vi "Send command.vi"(7 "Action":T2, 8 "error in (no error)":errorcluster, 9 "Set Values in":T1, 10 "d(0.0)":dbl, 11 "VISA resource":refnum<visa-resource-name>) -> (0 "error out":errorcluster, 1 "Set Values":T1, 3 "VISA resource out":refnum<visa-resource-name>)   [LabVIEW 2011]
doc: "Sends the actual command values, waits for the return strnig, but does not interprate it."
uses:
  Magna Commands.ctl
  Magna Configuration Values Set.ctl
  Magna PSU.lvlib
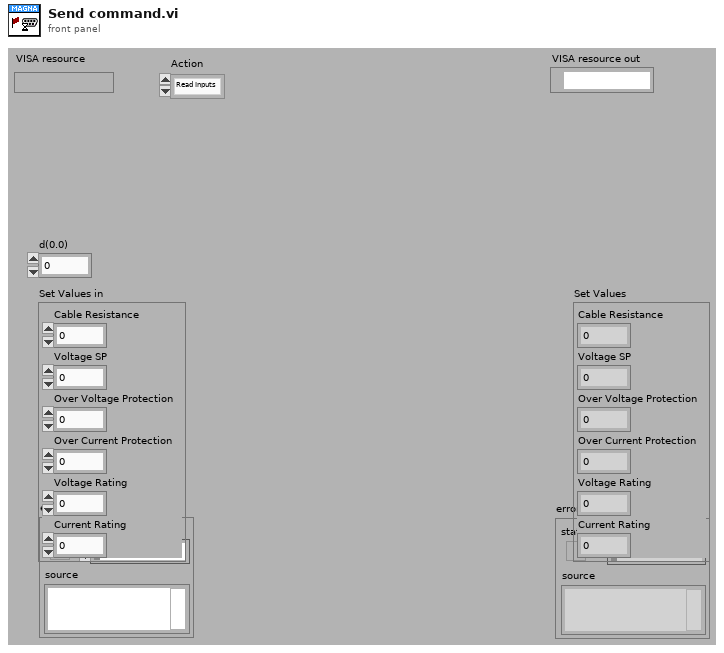
[diagram p1: front panel]
types:
  T1 = typedef "Magna Configuration Values Set.ctl" = cluster{"Cable Resistance":dbl, "Voltage SP":dbl, "Over Voltage Protection":dbl, "Over Current Protection":dbl, "Voltage Rating":dbl, "Current Rating":dbl}
  T2 = typedef "Magna Commands.ctl" = enum16{"Read Inputs", "HV ON", "HV OFF", "Set Resistance", "Set Head Voltage SP"}
  T3 = typedef "Options  All pages and custom.ctl" = cluster{"P 1 (App)":T4, "P 2":T5, "P 3":T6, "P 4":T9, "P 5":T14, "P 6 (Err)":T15, "P 7 (Expert)":T16, "P 8 (Depth)":T18, "C 1":T19, "C 2":T20}
  T4 = typedef "Options Page 1 (App).ctl" = cluster{"Result files":path, "PCP Interface":string, "Tractor/Stroker Interface":string, "Tractor Interface":string, "Modem Status Interface":string, "Audible Alarm":bool, "Force alarm on Technical":bool, "Force alarm on HH":bool, "Force alarm on LL":bool, "Force alarm on H":bool, "Force alarm on L":bool}
  T5 = typedef "Options Page 2.ctl" = cluster{"Solenoid & Relay latching time":u16, "Tractor relay 1":dbl, "Tractor relay 2":dbl, "Tractor Solenoid limit":dbl}
  T6 = typedef "Options Page 3.ctl" = cluster{"Min resistance":dbl, "Max resistance":dbl, "Head voltage range":T7, "Max voltage jump":dbl, "Maximum resistance change":dbl, "Start Telemetry Voltage":dbl, "Start Telemetry Timeout":dbl, "Start Motor Voltage":dbl, "Stop Motor Voltage":dbl, "Pass Mode Warning Voltage":dbl, "Relay Switch Voltage":dbl, "Relay Status Loss Voltage":dbl, "Samples to average":i32, "PSU type DO NOT USE":T8, "Magna OVP":dbl, "Magna Current Limit":dbl}
  T7 = typedef "PCP type List.ctl" = enum16{"0 - 350V", "0 - 450V", "0 - 600V"}
  T8 = typedef "PSU Type.ctl" = enum16{"Unipower", "Magna 8.3A", "Magna 12A", "None"}
  T9 = typedef "Options Page 4.ctl" = cluster{"Solenoid & Relay latching time":u16, "Stroker relay 1":dbl, "Stroker Relay 2":dbl, "Stroker Solenoid limit":dbl, "Force det.":T10, "Stroke force lim.":dbl, "Anchor Enabled Pressure":dbl, "Tacometer puls":dbl, "Default anchor behavior":T11, "Default stroker behavior":T12, "Default stroker force limit (tonne)":dbl, "Slips Size":T13}
  T10 = typedef "Stroke force selector.ctl" = enum16{"Stroke in = node 1", "Strok out = node 1"}
  T11 = typedef "Default anchor behavior.ctl" = enum16{"Do nothing", "Set Anchor", "Release Anchor"}
  T12 = typedef "Default stroker behavior.ctl" = enum16{"Do nothing", "Stop", "Go Out", "Go In"}
  T13 = typedef "Slips Type Radio.ctl" = enum32{"No Selection", "338 MRS", "3,9 MRS"}
  T14 = typedef "Options Page 5.ctl" = cluster{"Solenoid & Relay latching time":u16, "Driller relay 1":dbl, "Driller Relay 2":dbl, "Driller  Solenoid limit":dbl}
  T15 = typedef "Options Page 6 (Err).ctl" = cluster{"Error and event files":path}
  T16 = typedef "Options Page 7 (Expert).ctl" = cluster{"Show Debug":bool, "Log debug messages":bool, "Additional debug messages":bool, "Start Beagle with Simulator data":bool, "Workshop mode":bool, "Modem baud":u16, "enumCANCOM":bool, "Modem sim":T17, "Telemetry Timeout Disable":i32, "Buffer size":i32, "Upd regular data":bool, "Cable comp":cluster{"VMOD1 Voltage(V)":dbl, "VMOD2 Voltage(V)":dbl}}
  T17 = typedef "Modem simulation setup.ctl" = cluster{"Modem dealay sim":bool, "Sim baud Tx":u16, "Bit Error fraction Tx":dbl, "Sim baud Rx":u16, "Bit Error fraction Rx":dbl}
  T18 = typedef "Options Page 8 (Depth).ctl" = cluster{"Winch Spool Circumference":dbl, "Winch Pulses per Revolution":dbl, "Current Depth":dbl}
  T19 = typedef "Options Custom 1.ctl" = cluster{"Depth Updated":bool, "Depth Offset":dbl}
  T20 = typedef "Options Custom 2.ctl" = cluster{"Placeholder":bool}
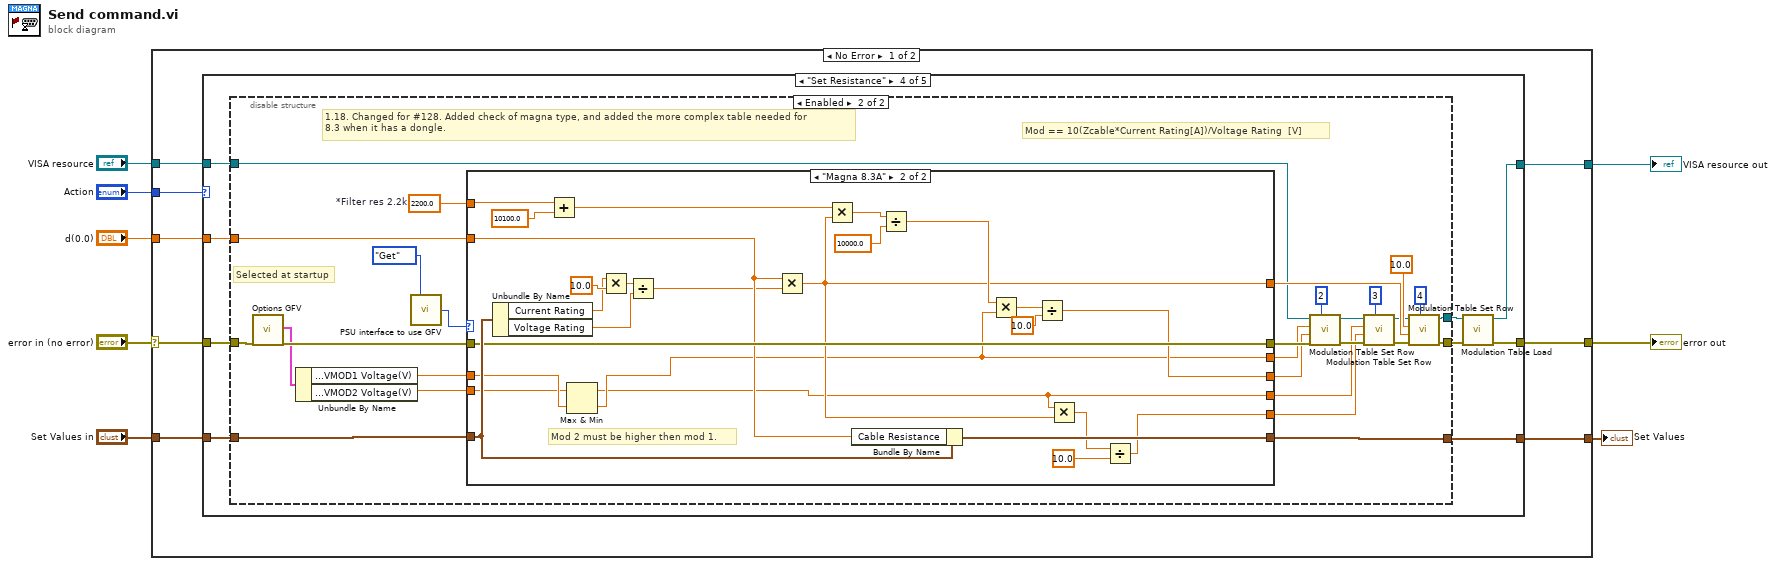
[diagram p0: block diagram]
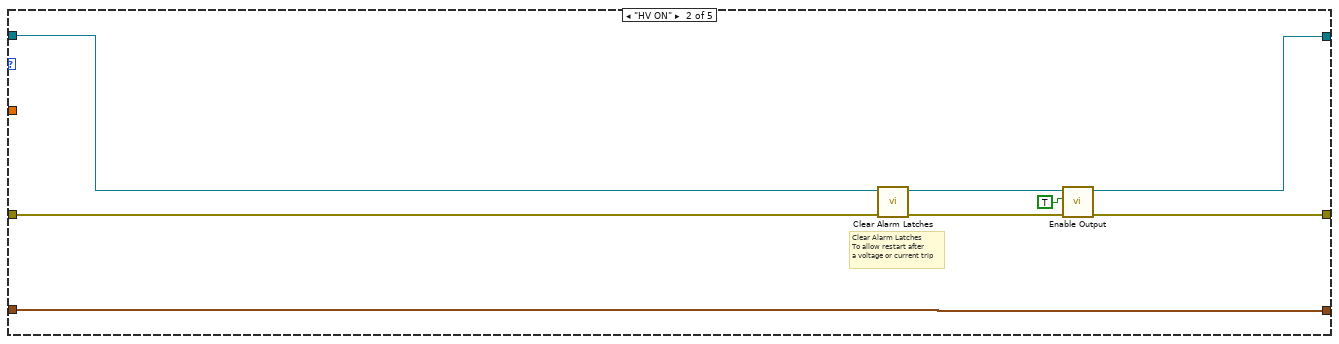
[diagram p3: hidden frame]
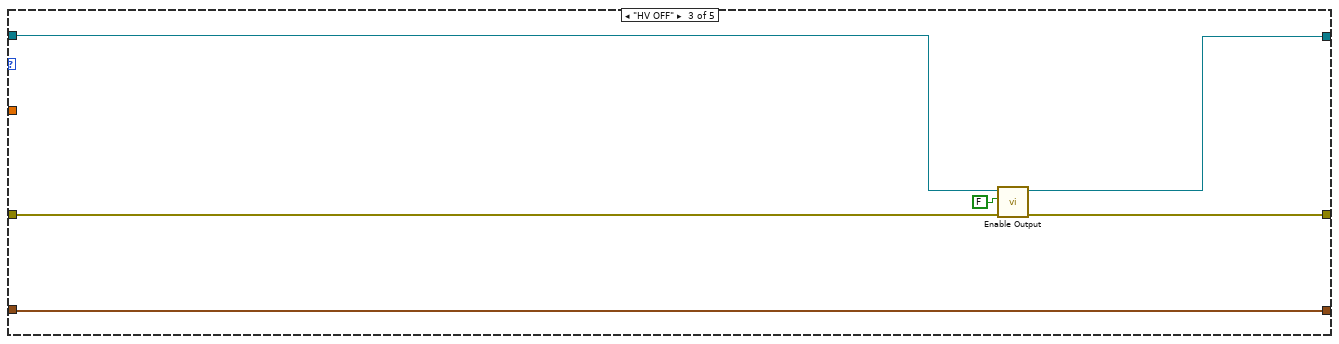
[diagram p4: hidden frame]
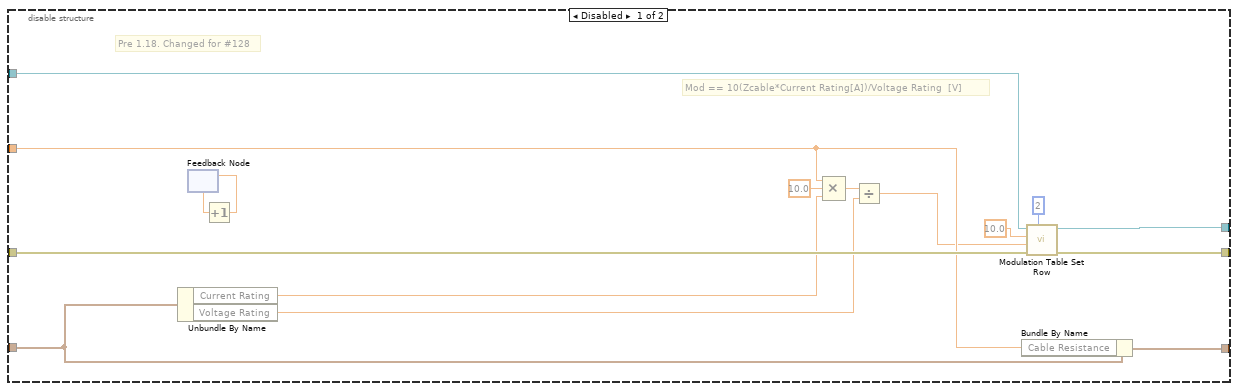
[diagram p5: hidden frame]
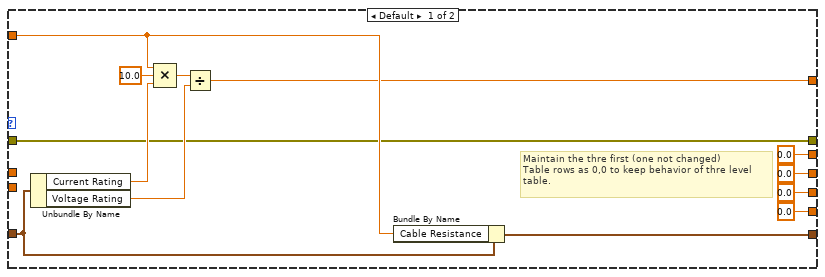
[diagram p6: hidden frame]
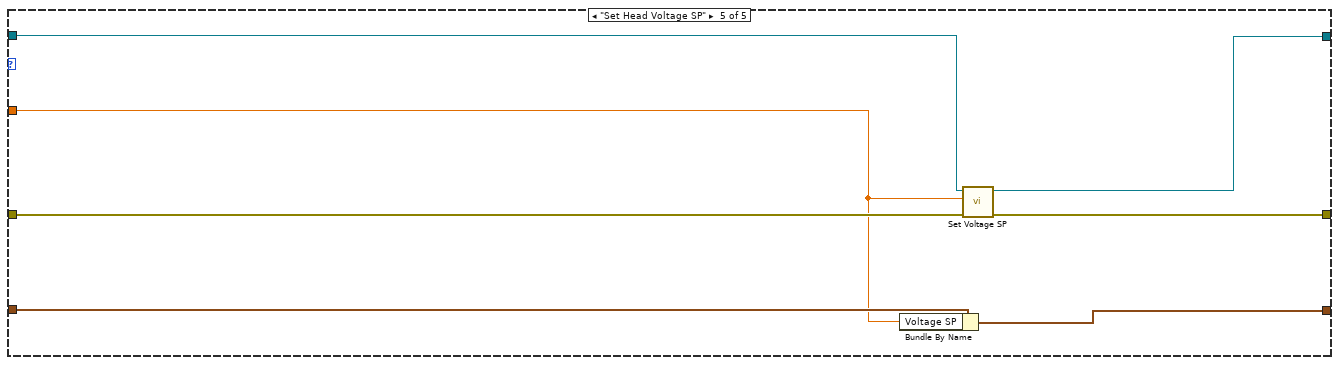
[diagram p7: hidden frame]
diagram:
  n1 = case shown="No Error" "error in (no error)" {
    selector: "error in (no error)" -> [w12 w134]
    tunnel: [w13 w134] -> w7
    tunnel: "VISA resource" -> [w15 w135]
    tunnel: [w14 w135] -> w5
    tunnel: "Action" -> [w16 _]
    tunnel: "d(0.0)" -> [w11 _]
    tunnel: [w10 w133] -> w2
    tunnel: "Set Values in" -> [w9 w133]
    frame No Error {
      n2 = case shown="\"Set Resistance\"" w16 {
        tunnel: w15 -> [w19 w23 w30 w41 w130]
        tunnel: [w19 w27 w33 w37 w129] -> w14
        tunnel: [w18 w25 w31 w36 w131] -> w13
        tunnel: w12 -> [w18 w22 w29 w42 w132]
        tunnel: w9 -> [w17 w24 w28 w35 w128]
        tunnel: w11 -> [_ _ _ w34 w126]
        tunnel: [w17 w24 w28 w40 w127] -> w10
        frame "Read Inputs", Default {
        }
        frame "HV ON" {
          # "Clear Alarm Latches\nTo allow restart after\na voltage or current trip"
          n3 = call "Clear Alarm Latches.vi"("error in (no error)"=w22, "VISA Refnum in"=w23) -> ("error out"=w21:errorcluster, "VISA Refnum out"=w20:refnum<visa-resource-name>)  [unwired: 8 in]
          n4 = call "Enable Output.vi"("error in (no error)"=w21, "Output Control"=TRUE, "VISA session"=w20) -> ("error out"=w25:errorcluster, "dup VISA session"=w27:refnum<visa-resource-name>)  [unwired: 7 in]
        }
        frame "HV OFF" {
          n5 = call "Enable Output.vi"("error in (no error)"=w29, "Output Control"=FALSE, "VISA session"=w30) -> ("error out"=w31:errorcluster, "dup VISA session"=w33:refnum<visa-resource-name>)  [unwired: 7 in]
        }
        frame "Set Resistance" {
          n6 = disable-structure shown="Enabled" {
            disable-tunnel: w42 -> [w56 w63]
            disable-tunnel: w41 -> [w55 w73]
            disable-tunnel: [w54 w84] -> w40
            disable-tunnel: [w51 w83] -> w39
            disable-tunnel: [w50 w82] -> w38
            disable-tunnel: w35 -> [w49 w81]
            disable-tunnel: w34 -> [w48 w80]
            frame Disabled {
              # "Pre 1.18. Changed for #128"
              # "Mod == 10(Zcable*Current Rating[A])/Voltage Rating  [V]"
              n7 = Unbundle By Name(w49) -> ("Current Rating"=w45:dbl, "Voltage Rating"=w43:dbl)
              n8 = feedback #1() -> (w52:dbl)  [unwired: 1 in]
              n9 = Increment(x=w52) -> (x+1=w53:dbl)
              n10 = feedback-in #1(w53) -> ()
              n11 = Compound Arithmetic op=MULTIPLY(w48, 10.0 ("y"), w45) -> (w46:dbl)
              n12 = Divide(x=w46, y=w43) -> (x/y=w44:dbl)
              n13 = Bundle By Name(cluster=w49, "Cable Resistance"=w48) -> (w54:T1)
              n14 = call "Modulation Table Set Row.vi"("Row"=i8 2, "error in (no error)"=w56, "Modulation Factor"=w44, "Modulation Voltage"=10.0, "VISA session in"=w55) -> ("error out"=w50:errorcluster, "VISA session out"=w51:refnum<visa-resource-name>)  [unwired: 5 in]
            }
            frame Enabled {
              w66 = 2200.0  # *Filter res 2.2k
              # "Selected at startup"
              # "1.18. Changed for #128. Added check of magna type, and added the more complex table needed for \n8.3 when it has a dongle."
              # "Mod == 10(Zcable*Current Rating[A])/Voltage Rating  [V]"
              n15 = call "Options GFV.vi"("error in (no error)"=w63) -> ("Options"=w61:T3, "error out"=w62:errorcluster)  [unwired: 16 in, 1 out]
              n16 = Unbundle By Name(w61) -> ("P 7 (Expert).Cable comp.VMOD1 Voltage(V)"=w60:dbl, "P 7 (Expert).Cable comp.VMOD2 Voltage(V)"=w59:dbl)
              n17 = call "PSU interface to use GFV.vi"("Action"=enum16{"Get", "Set"}."Get") -> ("PSU type  out"=w64:T8)  [unwired: 13 in, 1 out]
              n18 = case shown="\"Magna 8.3A\"" w64 {
                tunnel: [w99 w125] -> w84
                tunnel: w81 -> [w98 w124]
                tunnel: w80 -> [w97 w118]
                tunnel: [w92 w104] -> w79
                tunnel: w62 -> [w91 w119]
                tunnel: [w91 w119] -> w74
                tunnel: [0.0 ("Modulation Voltage") w100] -> w70
                tunnel: [0.0 ("Modulation Voltage") w105] -> w69
                tunnel: [0.0 ("Modulation Voltage") w102] -> w68
                tunnel: [0.0 ("Modulation Voltage") w109] -> w67
                tunnel: w60 -> [_ w103]
                tunnel: w59 -> [_ w101]
                tunnel: w66 -> [_ w117]
                frame Default {
                  # "Maintain the thre first (one not changed)\nTable rows as 0,0 to keep behavior of thre level \ntable."
                  n19 = Unbundle By Name(w98) -> ("Current Rating"=w94:dbl, "Voltage Rating"=w93:dbl)
                  n20 = Compound Arithmetic op=MULTIPLY(w97, 10.0 ("y"), w94) -> (w95:dbl)
                  n21 = Divide(x=w95, y=w93) -> (x/y=w92:dbl)
                  n22 = Bundle By Name(cluster=w98, "Cable Resistance"=w97) -> (w99:T1)
                }
                frame "Magna 8.3A" {
                  # "Mod 2 must be higher then mod 1."
                  n23 = Unbundle By Name(w124) -> ("Current Rating"=w121:dbl, "Voltage Rating"=w120:dbl)
                  n24 = Add(x=w117, y=10100.0) -> (x+y=w115:dbl)
                  n25 = Max & Min(x=w101, y=w103) -> (max(x,y)=w100:dbl, min(x,y)=w102:dbl)
                  n26 = Multiply(x=w121, y=10.0) -> (x*y=w122:dbl)
                  n27 = Divide(x=w122, y=w120) -> (x/y=w108:dbl)
                  n28 = Multiply(x=w118, y=w108) -> (x*y=w104:dbl)
                  n29 = Multiply(x=w115, y=w104) -> (x*y=w114:dbl)
                  n30 = Bundle By Name(cluster=w124, "Cable Resistance"=w118) -> (w125:T1)
                  n31 = Divide(x=w114, y=10000.0) -> (x/y=w112:dbl)
                  n32 = Multiply(x=w112, y=w102) -> (x*y=w111:dbl)
                  n33 = Divide(x=w111, y=10.0) -> (x/y=w109:dbl)
                  n34 = Multiply(x=w100, y=w104) -> (x*y=w106:dbl)
                  n35 = Divide(x=w106, y=10.0) -> (x/y=w105:dbl)
                }
              }
              n36 = call "Modulation Table Set Row.vi"("Row"=i8 2, "error in (no error)"=w74, "Modulation Factor"=w67, "Modulation Voltage"=w68, "VISA session in"=w73) -> ("error out"=w76:errorcluster, "VISA session out"=w72:refnum<visa-resource-name>)  [unwired: 5 in]
              n37 = call "Modulation Table Set Row.vi"("Row"=i8 3, "error in (no error)"=w76, "Modulation Factor"=w69, "Modulation Voltage"=w70, "VISA session in"=w72) -> ("error out"=w75:errorcluster, "VISA session out"=w71:refnum<visa-resource-name>)  [unwired: 5 in]
              n38 = call "Modulation Table Set Row.vi"("Row"=i8 4, "error in (no error)"=w75, "Modulation Factor"=w79, "Modulation Voltage"=10.0, "VISA session in"=w71) -> ("error out"=w82:errorcluster, "VISA session out"=w83:refnum<visa-resource-name>)  [unwired: 5 in]
            }
          }
          n39 = call "Modulation Table Load.vi"("error in (no error)"=w38, "VISA session in"=w39) -> ("error out"=w36:errorcluster, "VISA session out"=w37:refnum<visa-resource-name>)  [unwired: 8 in]
        }
        frame "Set Head Voltage SP" {
          n40 = Bundle By Name(cluster=w128, "Voltage SP"=w126) -> (w127:T1)
          n41 = call "Set Voltage SP.vi"("error in (no error)"=w132, "Voltage SP"=w126, "VISA session"=w130) -> ("error out"=w131:errorcluster, "dup VISA session"=w129:refnum<visa-resource-name>)  [unwired: 7 in]
        }
      }
    }
    frame Error {
    }
  }
  "error out" <- w7
  "VISA resource out" <- w5
  "Set Values" <- w2
